vi "Exercise5_2.vi"() -> ()   [LabVIEW 2015]
doc: "This VI demonstrates how the order in which you apply transformations to an object in a 3D scene affects the object's position and orientation within the scene. \n\n<b>Rotate then Translate:</b>\nIf you apply a rotation to an object as the first transformation, the object rotates around its parent's axis, which exists in spatially the same place as the object's own axis. Regardless of what transformations follow the rotation, the object appears to rotate around its own axis. If you apply a translation after the rotation, the object appears offset from its parent and still spinning around its own axis.\n\n<b>Translate then Rotate:</b>\nIf you apply a translation to an object as the first transformation, the object still appears offset from its parent. However, if you then apply a rotation to the object, the object rotates around its parent by the angle you specify with the Translate Object VI."
panel:
  out "error out":errorcluster
  out "RPY":cluster{"roll":dbl, "pitch":dbl, "yaw":dbl}
  out "euler ZYZ":T1
  out "Orientation matrix":dbl[][](array[numeric])
  in  "XYZ":dbl[](array[numeric]) format="%0.2f"
  in  "a":dbl[](array[numeric]) format="%0.2f"
  in  "o":dbl[](array[numeric]) format="%0.2f"
  in  "Stop":bool
  out "3D Picture":refnum<vi>(3d-picture)
  # "Position and Orientation POSE"
  # "XYZ --> Mobile frame\nZYX --> Fixed frame"
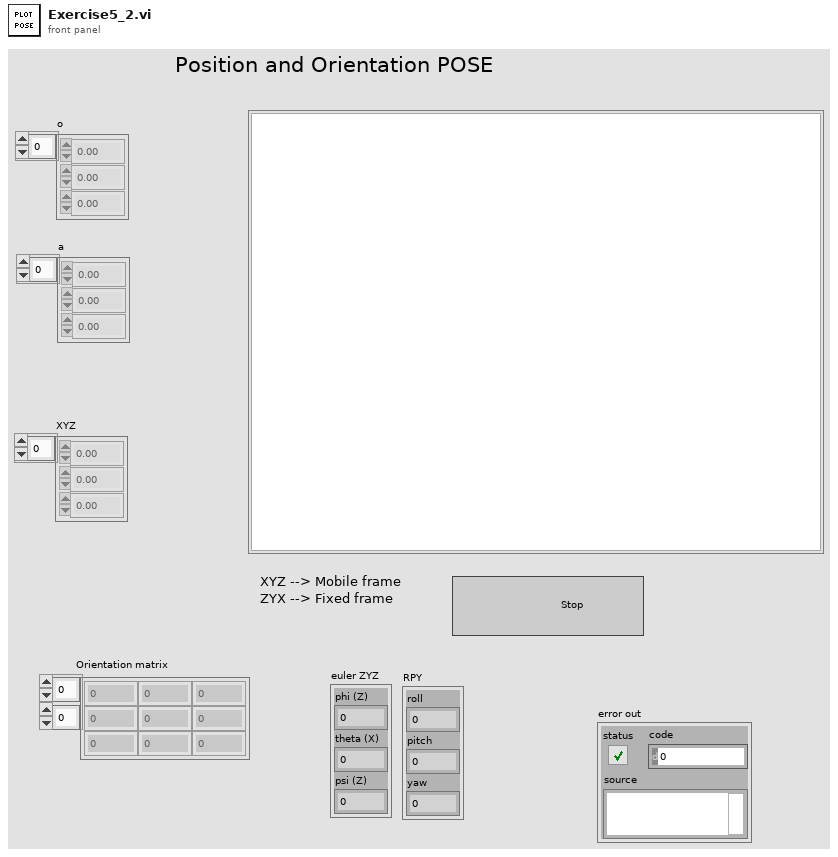
[diagram p1: front panel]
types:
  T1 = cluster{"phi (Z)":dbl, "theta (X)":dbl, "psi (Z)":dbl}
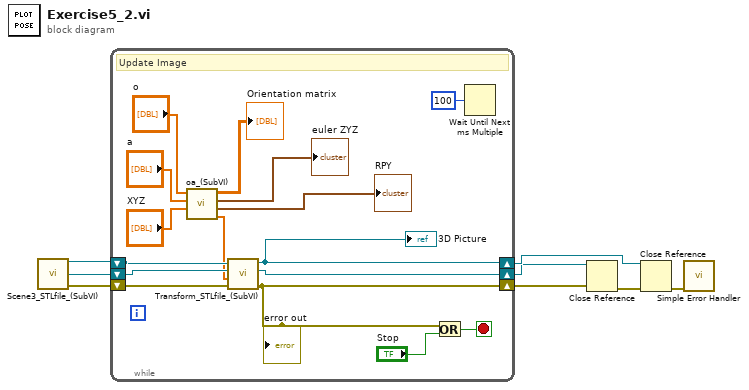
[diagram p0: block diagram]
diagram:
  n1 = call "Scene3_STLfile_(SubVI).vi"() -> ("error out"=w1:errorcluster, "New Object Out"=w2:refnum<vi>, "SceneObject out"=w3:refnum<vi>)  [unwired: 9 in]
  n2 = while {
    shift-right: [w16] -> w7
    shift-left: w1 -> [w19]
    shift-right: [w17] -> w4
    shift-left: w2 -> [w20]
    shift-right: [w18] -> w8
    shift-left: w3 -> [w21]
    stop <- w23 stop-if-true
    # "Update Image"
    n3 = call "oa_(SubVI).vi"("XYZ"="XYZ", "a"="a", "o"="o") -> ("POSE"=w15:dbl[], "RPY"=→"RPY":cluster{"roll":dbl, "pitch":dbl, "yaw":dbl}, "euler ZYZ"=→"euler ZYZ":T1, "Array"=→"Orientation matrix":dbl[][])  [unwired: 5 in]
    n4 = call "Transform_STLfile_(SubVI).vi"("error in (no error)"=w19, "POSE"=w15, "New Object In"=w20, "SceneObject In"=w21) -> ("error out"=w16:errorcluster, "New Object out"=w17:refnum<vi>, "SceneObject Out"=w18:refnum<vi>)  [unwired: 5 in]
    "3D Picture" <- w18
    "error out" <- w16
    n5 = Or(x=w16, y="Stop") -> (x .or. y?=w23:bool)
    n6 = Wait Until Next ms Multiple(millisecond multiple=u32 100 ("milliseconds to wait")) -> ()  [unwired: 1 out]
  }
  n7 = Close Reference(reference=w4, error in (no error)=w7) -> (error out=w5:errorcluster)
  n8 = Close Reference(reference=w8, error in (no error)=w5) -> (error out=w6:errorcluster)
  n9 = call <vilib>:"Simple Error Handler.vi"("error in (no error)"=w6) -> ()  [unwired: 4 in, 5 out]
